vi "main.vi"() -> ()   [LabVIEW 2017]
uses:
  <vilib>/express/express arith-compare/Formula/XNode/ExpressFormulaBlockNode.xnode
  <vilib>/myRIO/Express VI/Onboard Devices/LED/LED Express VI.xnode
  <vilib>/myRIO/Instrument Drivers/Onboard IO/DIO/typedefs/DIO Reference.ctl
  <vilib>/myRIO/Instrument Drivers/Onboard IO/DIO/DIO.lvlib
  <vilib>/myRIO/Common/Instrument Driver Framework/myRIO v1.0/DIO/typedefs/DIO Channels List.ctl
  <vilib>/myRIO/Common/Instrument Driver Framework/myRIO v1.0/DIO/typedefs/DIO Channels Enum.ctl
  <vilib>/myRIO/Common/Instrument Driver Framework/Utilities/typedefs/myRIO Generic Hardware Reference.ctl
  <vilib>/myRIO/Common/Instrument Driver Framework/Utilities/typedefs/myRIO v1.0 Reference.ctl
  <vilib>/myRIO/Common/Instrument Driver Framework/Utilities/typedefs/Generic FPGA Reference.ctl
  <vilib>/myRIO/Common/Instrument Driver Framework/Utilities/typedefs/Hardware Version Enum.ctl
  <vilib>/myRIO/Instrument Drivers/Onboard IO/DIO/vis/Write.vi
  <vilib>/myRIO/Instrument Drivers/Onboard IO/DIO/vis/myRIO DIO Open.xnode
  <vilib>/userdefined/High Color/nirio_resource_hc.ctl
  <vilib>/myRIO/Common/Instrument Driver Framework/myRIO v1.0/DIO/vis/myRIO v1.1 Open DIO.vi
  <vilib>/myRIO/Common/Instrument Driver Framework/Utilities/vis/Is FPGA Ref Available.vi
panel:
  out "output array":dbl[](array[numeric])
  out "camera CCW?":bool=TRUE
  out "turn Number":i32
  in  "goal Y":dbl=100.0
  in  "goal X":dbl=144.0
  in  "distanceAllowValue":dbl
  in  "Coordinate":dbl[][](array[numeric])=[[30.0, 220.0], [230.0, 230.0], [225.0, 50.0]]
  out "now Y":dbl
  out "now X":dbl
  out "goal Distance":dbl
  out "robot Direction":dbl
  out "goal Direaction":dbl
  out "last Y":dbl
  out "last X":dbl
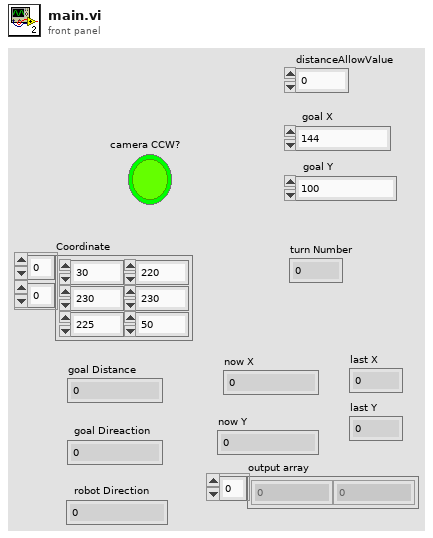
[diagram p1: front panel]
types:
  T1 = typedef "DIO.lvlib/DIO Reference.ctl" = cluster{"myRIO Reference":T2, "DIO Channels List":T6}
  T2 = typedef "myRIO Generic Hardware Reference.ctl" = cluster{"myRIO Model":T3, "myRIO Hardware Reference":T4}
  T3 = typedef "Hardware Version Enum.ctl" = enum16{"Unknown", "myRIO-1900", "myRIO-1950", "roboRIO", "NI ELVIS RIO CM"}
  T4 = typedef "myRIO v1.0 Reference.ctl" = cluster{"Generic FPGA Reference":T5, "Allow multiple opens":bool}
  T5 = typedef "Generic FPGA Reference.ctl" = refnum<k20>
  T6 = typedef "DIO Channels List.ctl" = T7[]
  T7 = typedef "DIO Channels Enum.ctl" = enum16{"Not Connected", "C/DIO0", "C/DIO1", "C/DIO2", "C/DIO3", "C/DIO4", "C/DIO5", "C/DIO6", "C/DIO7", "A/DIO0", "A/DIO1", "A/DIO2", "A/DIO3", "A/DIO4", "A/DIO5", "A/DIO6", "A/DIO7", "A/DIO8", "A/DIO9", "A/DIO10", "A/DIO11", "A/DIO12", "A/DIO13", "A/DIO14", "A/DIO15", "B/DIO0", "B/DIO1", "B/DIO2", "B/DIO3", "B/DIO4", "B/DIO5", "B/DIO6", "B/DIO7", "B/DIO8", "B/DIO9", "B/DIO10", "B/DIO11", "B/DIO12", "B/DIO13", "B/DIO14", "B/DIO15", "LED0", "LED1", "LED2", "LED3", "Button0", "DIO/DIO0", "DIO/DIO1", "DIO/DIO2", "DIO/DIO3", "DIO/DIO4", "DIO/DIO5", "DIO/DIO6", "DIO/DIO7", "DIO/DIO8", "DIO/DIO9", "SPI/CS0", "SPI/CS1", "SPI/CS2", "SPI/CS3", "LED RADIO (Green)", "LED RADIO (Red)", "LED COMM (Green)", "LED COMM (Red)", "LED MODE (Green)", "LED MODE (Red)"}
  T8 = typedef "nirio_resource_hc.ctl" = tag
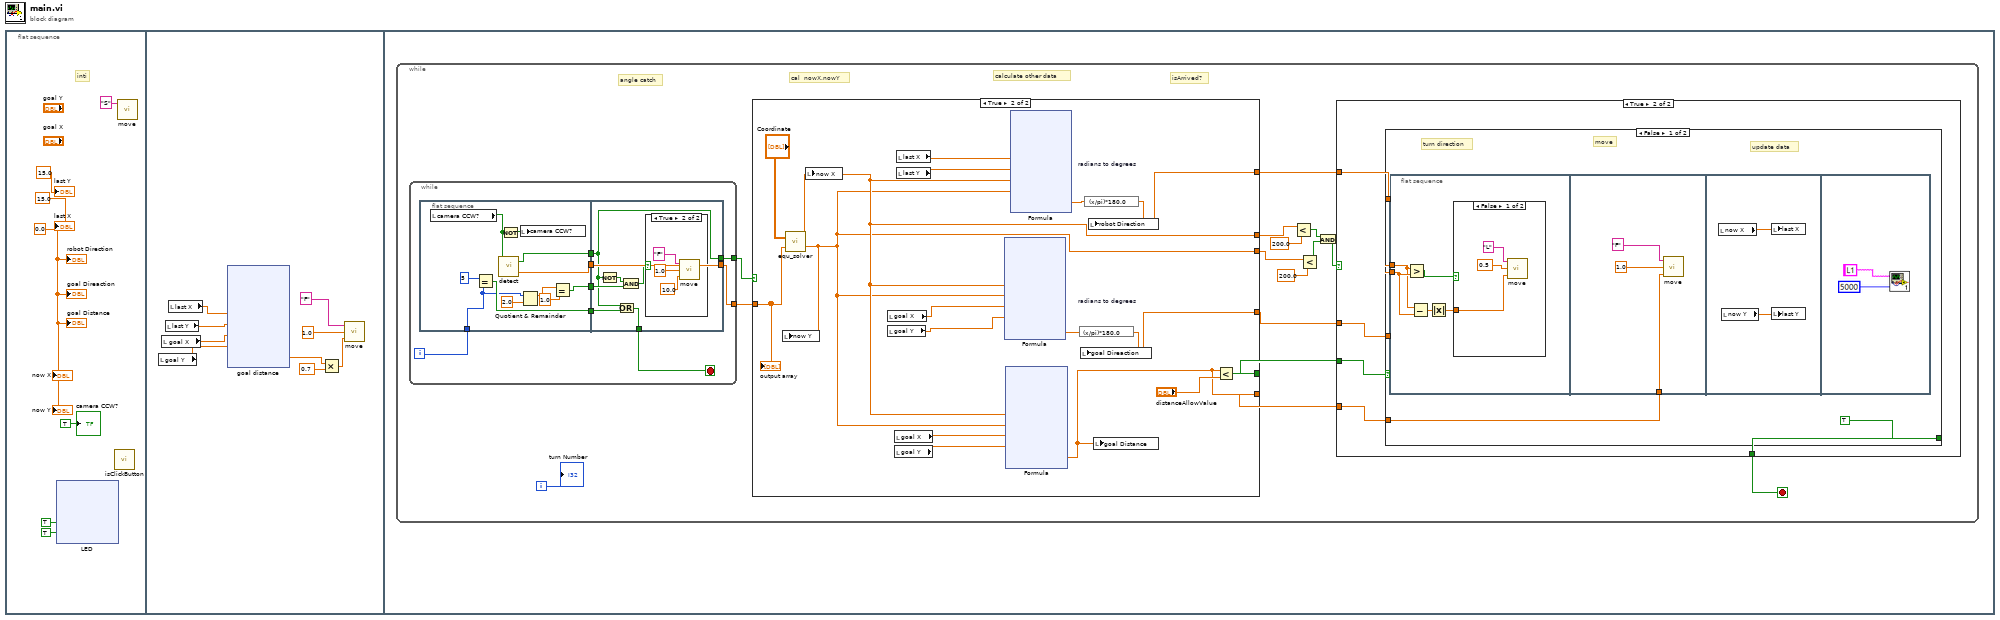
[diagram p0: block diagram]
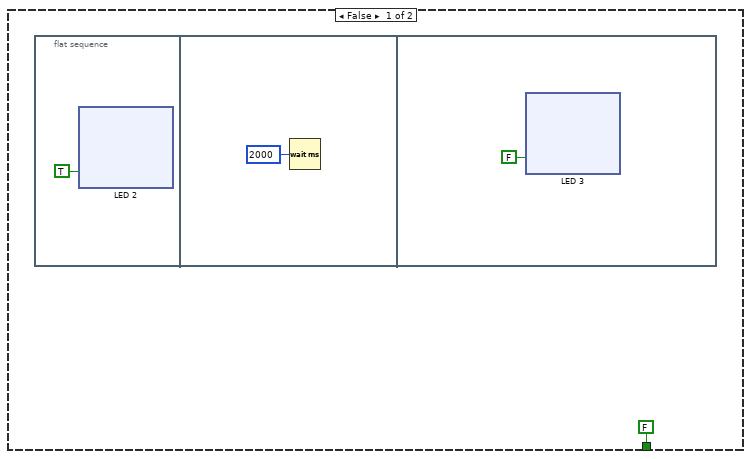
[diagram p2: hidden frame]
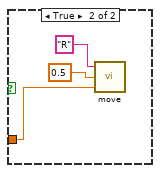
[diagram p3: hidden frame]
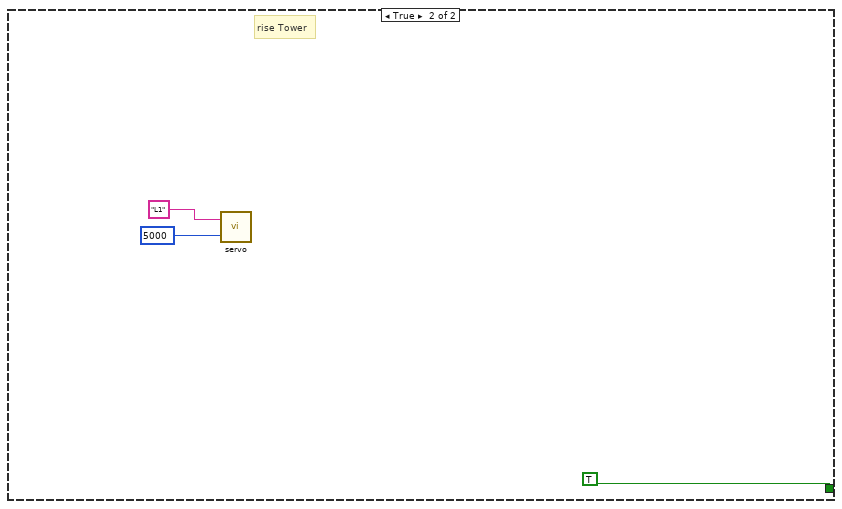
[diagram p4: hidden frame]
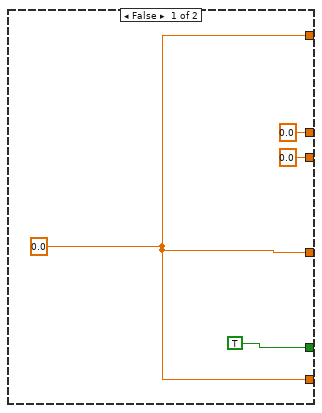
[diagram p5: hidden frame]
diagram:
  n1 = flat-sequence {
    frame #0 {
      w7 = 0.0 ("robot Direction")
      # "inti"
      n2 = xnode "LED"("LED2"=TRUE ("LED0"), "LED3"=TRUE ("LED2")) -> ()  [unwired: 1 in, 1 out]
      n3 = call "isClickButton.vi"() -> ()  [unwired: 1 in]
      n4 = call "move.vi"("mode"="S") -> ()  [unwired: 2 in]
      "last X" <- 15.0
      "last Y" <- 15.0
      "goal Direaction" <- w7
      "robot Direction" <- w7
      "goal Distance" <- w7
      "now X" <- w7
      "now Y" <- w7
      "camera CCW?" <- TRUE ("Boolean")
    }
    frame #1 {
      n5 = local read "goal Y"() -> (w50:dbl)
      n6 = local read "goal X"() -> (w49:dbl)
      n7 = local read "last Y"() -> (w48:dbl)
      n8 = local read "last X"() -> (w47:dbl)
      n9 = xnode "goal distance"("nowX"=w47, "nowY"=w48, "goalX"=w49, "goalY"=w50) -> ("Result"=w45:dbl)  [unwired: 1 in, 1 out]
      n10 = Multiply(x=w45, y=0.7) -> (x*y=w44:dbl)
      n11 = call "move.vi"("value( disatance or angle)"=w44, "Speed precent"=1.0, "mode"="F") -> ()
    }
    frame #2 {
      n12 = while {
        i -> [w80]
        stop <- w79 stop-if-true
        # "isArrived?"
        # "cal  nowX,nowY"
        # "angle catch"
        # "calculate other data"
        n13 = while {
          tunnel: [w254] -> w76
          tunnel: [w247] -> w74
          i -> [w253]
          stop <- w249 stop-if-true
          n14 = flat-sequence {
            tunnel: w253 -> [w256]
            tunnel: [w263] -> w252
            tunnel: [w261] -> w251
            tunnel: [w260] -> w250
            tunnel: [w255] -> w248
            tunnel: [w272] -> w254
            tunnel: w252 -> [w272]
            tunnel: w251 -> [w266]
            tunnel: w250 -> [w271]
            tunnel: [w270] -> w249
            tunnel: w248 -> [w268]
            tunnel: [w266] -> w247
            frame #0 {
              n15 = local read "camera CCW?"() -> (w264:bool)
              n16 = Equal?(x=5, y=w256) -> (x = y?=w260:bool)
              n17 = call "detect.vi"("rotate\nCCW?"=w264) -> ("output array"=w263:dbl[], "isSuccess?"=w261:bool)  [unwired: 1 in]
              n18 = Not(x=w264) -> (.not. x?=w265:bool)
              n19 = local write "camera CCW?"(w265) -> ()
              n20 = Quotient & Remainder(x=w256, y=2.0) -> (x-y*floor(x/y)=w259:dbl)  [unwired: 1 out]
              n21 = Equal?(x=w259, y=1.0) -> (x = y?=w255:bool)
            }
            frame #1 {
              n22 = Not(x=w266) -> (.not. x?=w269:bool)
              n23 = Or(x=w266, y=w271) -> (x .or. y?=w270:bool)
              n24 = And(x=w269, y=w268) -> (x .and. y?=w267:bool)
              n25 = case shown="True" w267 {
                frame False {
                }
                frame True {
                  n26 = call "move.vi"("value( disatance or angle)"=10.0, "Speed precent"=1.0, "mode"="F" ("String")) -> ()
                }
              }
            }
          }
        }
        n27 = case shown="True" w74 {
          tunnel: [TRUE w200] -> w81
          tunnel: [w186 w194] -> w78
          tunnel: [w186 w192] -> w77
          tunnel: w76 -> [_ w191]
          tunnel: [w186 w190] -> w75
          tunnel: [0.0 ("now X") w189] -> w73
          tunnel: [0.0 ("now Y") w188] -> w70
          frame False {
            w186 = 0.0 ("Result")
          }
          frame True {
            n28 = call "equ_solver.vi"("theta"=w191, "Coordination"="Coordinate") -> ("now Y"=w188:dbl, "now X"=w189:dbl)
            n29 = local write "now Y"(w188) -> ()
            n30 = local write "now X"(w189) -> ()
            n31 = local read "goal X"() -> (w196:dbl)
            n32 = local read "goal Y"() -> (w197:dbl)
            n33 = local read "goal X"() -> (w199:dbl)
            n34 = local read "goal Y"() -> (w198:dbl)
            n35 = local read "last X"() -> (w204:dbl)
            n36 = local read "last Y"() -> (w203:dbl)
            n37 = xnode "Formula"("nowX"=w189, "nowY"=w188, "goalX"=w196, "goalY"=w197) -> ("Result"=w195:dbl)  [unwired: 1 in, 1 out]
            n38 = xnode "Formula"("nowX"=w189, "nowY"=w188, "goalX"=w199, "goalY"=w198) -> ("Result"=w190:dbl)  [unwired: 1 in, 1 out]
            n39 = xnode "Formula"("lastX"=w204, "lastY"=w203, "nowX"=w189, "nowY"=w188) -> ("Result"=w193:dbl)  [unwired: 1 in, 1 out]
            n40 = expression code="(x/pi)*180.0" "radians to degrees"(w195) -> (w194:dbl)
            n41 = local write "goal Direaction"(w194) -> ()
            n42 = expression code="(x/pi)*180.0" "radians to degrees"(w193) -> (w192:dbl)
            n43 = local write "robot Direction"(w192) -> ()
            n44 = local write "goal Distance"(w190) -> ()
            n45 = Less?(x=w190, y="distanceAllowValue") -> (x < y?=w200:bool)
            "output array" <- w191
          }
        }
        n46 = Less?(x=w73, y=200.0) -> (x < y?=w69:bool)
        n47 = Less?(x=w70, y=200.0) -> (x < y?=w68:bool)
        n48 = And(x=w69, y=w68) -> (x .and. y?=w67:bool)
        n49 = case shown="True" w67 {
          tunnel: w81 -> [_ w160]
          tunnel: [FALSE w159] -> w79
          tunnel: w78 -> [_ w158]
          tunnel: w77 -> [_ w157]
          tunnel: w75 -> [_ w156]
          frame False {
            n50 = flat-sequence {
              frame #0 {
                n51 = xnode "LED 2"("LED1"=TRUE) -> ()  [unwired: 1 in, 1 out]
              }
              frame #1 {
                n52 = Wait (ms)(milliseconds to wait=u32 2000) -> ()  [unwired: 1 out]
              }
              frame #2 {
                n53 = xnode "LED 3"("LED1"=FALSE) -> ()  [unwired: 1 in, 1 out]
              }
            }
          }
          frame True {
            n54 = case shown="False" w160 {
              tunnel: w157 -> [w163 _]
              tunnel: w158 -> [w162 _]
              tunnel: [TRUE TRUE] -> w159
              tunnel: w156 -> [w161 _]
              frame False {
                # "update data"
                # "move"
                # "turn direction"
                n55 = flat-sequence {
                  tunnel: w163 -> [w167]
                  tunnel: w162 -> [w168]
                  tunnel: w161 -> [w178]
                  frame #0 {
                    n56 = Greater?(x=w167, y=w168) -> (0:w169:bool)
                    n57 = Subtract(x=w167, y=w168) -> (x-y=w166:dbl)
                    n58 = Absolute Value(x=w166) -> (abs(x)=w165:dbl)
                    n59 = case shown="False" w169 {
                      tunnel: w165 -> [w170 w173]
                      frame False {
                        n60 = call "move.vi"("value( disatance or angle)"=w170, "Speed precent"=0.5, "mode"="L" ("String")) -> ()
                      }
                      frame True {
                        n61 = call "move.vi"("value( disatance or angle)"=w173, "Speed precent"=0.5, "mode"="R" ("String")) -> ()
                      }
                    }
                  }
                  frame #1 {
                    n62 = call "move.vi"("value( disatance or angle)"=w178, "Speed precent"=1.0, "mode"="F" ("String")) -> ()
                  }
                  frame #2 {
                    n63 = local read "now X"() -> (w179:dbl)
                    n64 = local read "now Y"() -> (w180:dbl)
                    n65 = local write "last X"(w179) -> ()
                    n66 = local write "last Y"(w180) -> ()
                  }
                  frame #3 {
                  }
                }
              }
              frame True {
                # "rise Tower"
                n67 = call "servo.vi"("milliseconds to wait"=u32 5000, "mode"="L1") -> ()  [unwired: 1 in]
              }
            }
          }
        }
        "turn Number" <- w80
      }
    }
  }
